vi "main.vi"() -> ()   [LabVIEW 2023]
uses:
  #typedef_info.ctl
  #typdef_state.ctl
panel:
  out "Info":T1
  in  "Stop":bool
  in  "Run Cleaning":bool
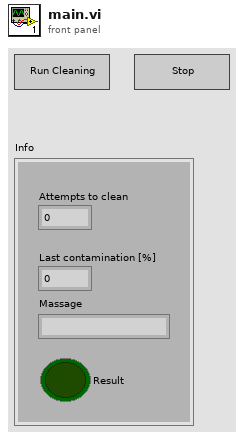
[diagram p1: front panel]
types:
  T1 = typedef "#typedef_info.ctl" = cluster{"Last contamination [%]":dbl, "Attempts to clean":i32, "Massage":string, "Result":bool}
  T2 = typedef "#typdef_state.ctl" = enum16{"Application Error", "Inicializing", "Idling", "Cleaning", "Stop"}
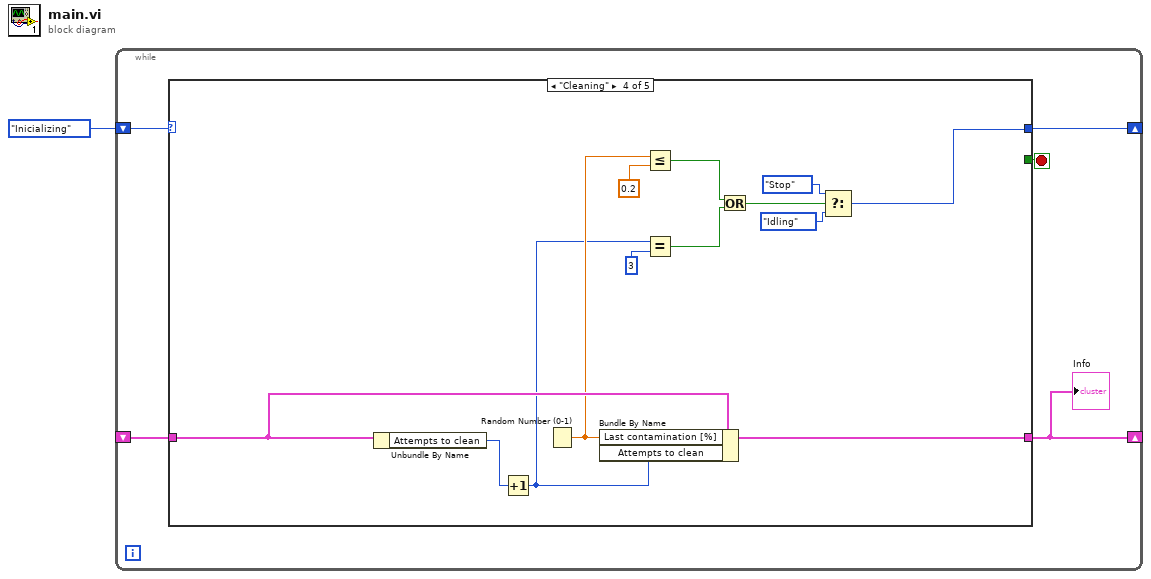
[diagram p0: block diagram]
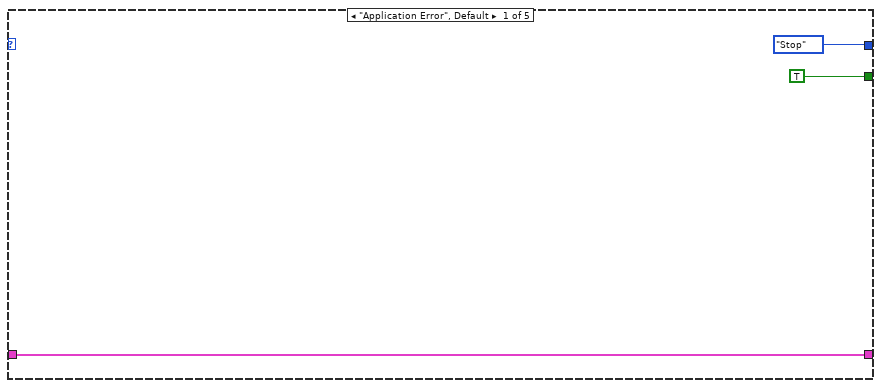
[diagram p2: hidden frame]
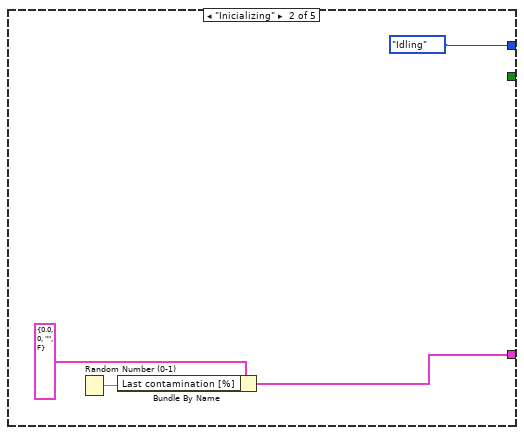
[diagram p3: hidden frame]
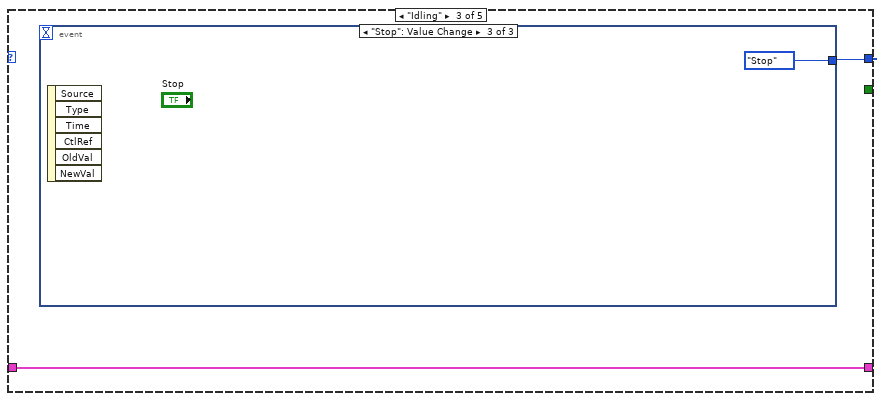
[diagram p4: hidden frame]
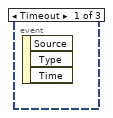
[diagram p5: hidden frame]
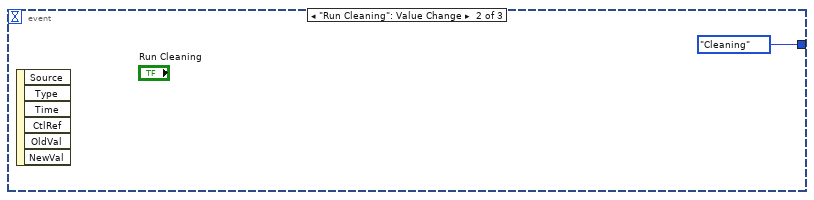
[diagram p6: hidden frame]
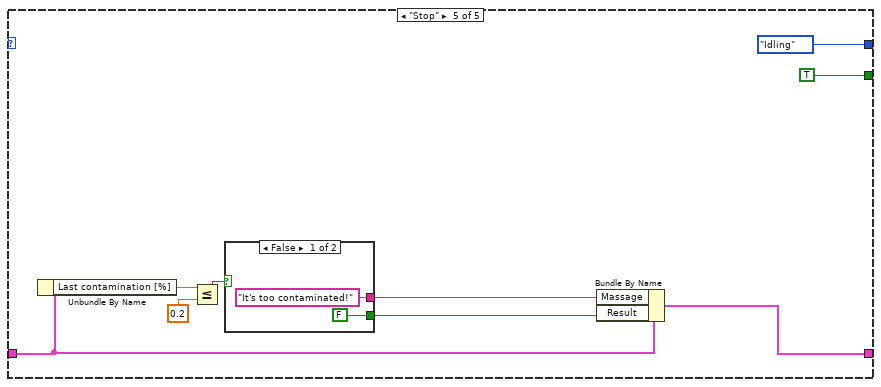
[diagram p7: hidden frame]
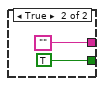
[diagram p8: hidden frame]
diagram:
  n1 = while {
    shift-right: [w4] -> _
    shift-left: #typdef_state."Inicializing" ("State") -> [w6]
    shift-right: [w3] -> _
    shift-left: _ -> [w5]
    stop <- w2 stop-if-true
    n2 = case shown="\"Cleaning\"" w6 {
      tunnel: [w9 w11 w15 w28 w31] -> w3
      tunnel: w5 -> [w9 _ w15 w29 w37]
      tunnel: [#typdef_state."Stop" ("State") #typdef_state."Idling" ("State") w14 w20 #typdef_state."Idling" ("State")] -> w4
      tunnel: [TRUE _ _ _ TRUE] -> w2
      frame "Application Error", Default {
      }
      frame "Inicializing" {
        n3 = Random Number (0-1)() -> (number: 0 to 1=w13:dbl)
        n4 = Bundle By Name(cluster=T1 {"Last contamination [%]"=0.0, "Attempts to clean"=0, "Massage"="", "Result"=FALSE} ("Info 2"), "Last contamination [%]"=w13) -> (w11:T1)
      }
      frame "Idling" {
        n5 = event shown="[2] \"Stop\": Value Change" {
          selector: _ -> [_ _ _]
          dyn-events: _ -> [_ _ _]
          timeout: _ -> [_ _ _]
          tunnel: [_ #typdef_state."Cleaning" ("State") #typdef_state."Stop" ("State")] -> w14
          event Timeout {
            n6 = event-data() -> ()  [unwired: 1 in, 3 out]
          }
          event "Run Cleaning": Value Change {
            n7 = event-data() -> ()  [unwired: 1 in, 6 out]
          }
          event "Stop": Value Change {
            n8 = event-data() -> ()  [unwired: 1 in, 6 out]
          }
        }
      }
      frame "Cleaning" {
        n9 = Unbundle By Name(w29) -> ("Attempts to clean"=w30:i32)
        n10 = Increment(x=w30) -> (x+1=w24:i32)
        n11 = Random Number (0-1)() -> (number: 0 to 1=w27:dbl)
        n12 = Bundle By Name(cluster=w29, "Last contamination [%]"=w27, "Attempts to clean"=w24) -> (w28:T1)
        n13 = Less Or Equal?(x=w27, y=0.2) -> (x <= y?=w23:bool)
        n14 = Equal?(x=w24, y=3) -> (x = y?=w22:bool)
        n15 = Or(x=w23, y=w22) -> (x .or. y?=w21:bool)
        n16 = Select(t=#typdef_state."Stop" ("State"), s=w21, f=#typdef_state."Idling" ("State")) -> (s? t:f=w20:T2)
      }
      frame "Stop" {
        n17 = Unbundle By Name(w37) -> ("Last contamination [%]"=w35:dbl)
        n18 = Less Or Equal?(x=w35, y=0.2) -> (x <= y?=w36:bool)
        n19 = case shown="False" w36 {
          tunnel: ["It's too contaminated!" ""] -> w33
          tunnel: [FALSE TRUE] -> w32
          frame False {
          }
          frame True {
          }
        }
        n20 = Bundle By Name(cluster=w37, "Massage"=w33, "Result"=w32) -> (w31:T1)
      }
    }
    "Info" <- w3
  }
